vi "End Undo Transaction.vi"(7 "Transaction? (TRUE)":bool, 8 "error in (no error)":errorcluster, 11 "VI in":refnum<vi>) -> (0 "error out":errorcluster, 3 "VI out":refnum<vi>)   [LabVIEW 2013]
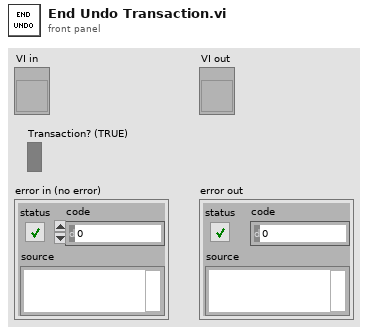
[diagram p1: front panel]
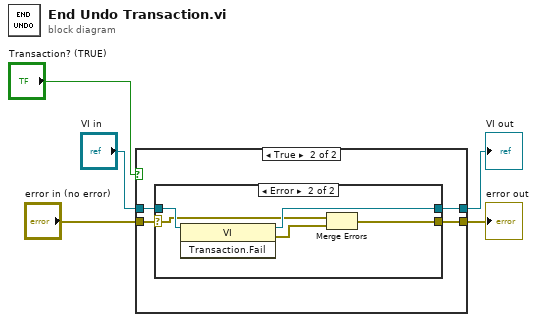
[diagram p0: block diagram]
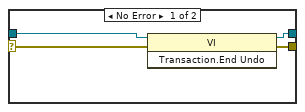
[diagram p3: hidden frame]
diagram:
  n1 = case shown="True" "Transaction? (TRUE)" {
    tunnel: "error in (no error)" -> [w6 w11]
    tunnel: [w6 w10] -> w2
    tunnel: [w7 w9] -> w3
    tunnel: "VI in" -> [w7 w8]
    frame False {
    }
    frame True {
      n2 = case shown="Error" w11 {
        selector: w11 -> [w14 w18]
        tunnel: w8 -> [w15 w20]
        tunnel: [w13 w19] -> w9
        tunnel: [w12 w16] -> w10
        frame No Error {
          # "If no errors occur, call the End Undo method to commit the transaction."
          n3 = invoke class="VI" method="Transaction.End Undo"(reference=w15, error in=w14) -> (reference out=w13:refnum<vi>, error out=w12:errorcluster)  [unwired: 1 in, 1 out]
        }
        frame Error {
          # "If errors do occur, call the Fail method to revert the VI to its state prior to the start of the Undo transaction.  The error in terminal of the Fail method is left unwired so the Fail method will always execute to revert the change."
          n4 = invoke class="VI" method="Transaction.Fail"(reference=w20) -> (reference out=w19:refnum<vi>, error out=w17:errorcluster)  [unwired: 2 in, 1 out]
          n5 = Merge Errors(w18, w17) -> (w16:errorcluster)
        }
      }
    }
  }
  "VI out" <- w3
  "error out" <- w2
